vi "GUI.vi"() -> ()   [LabVIEW 2021]
doc: "The UDP protocol differs from TCP in that there is no error-checking with the packets of information that are sent, and thus no guarantee whatsoever that an intended recipient will actually receive a given piece of data.\n\nUDP does offer the ability to \"broadcast\" data across a network--simply specify an IP Address of all ones (255.255.255.255) to attempt to broadcast information network-wide. Keep in mind that routers and other network hardware will generally refuse to forward the broadcast beyond certain points, so the extent of the broadcast will in practice be limited."
panel:
  out "Waveform Chart":i32(graph)
  out "data out":string
  out "tx":i32
  in  "Stop":bool
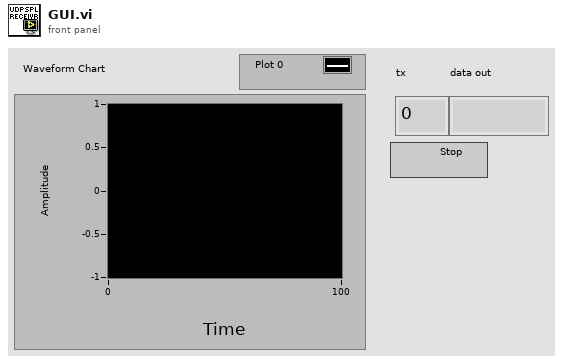
[diagram p1: front panel]
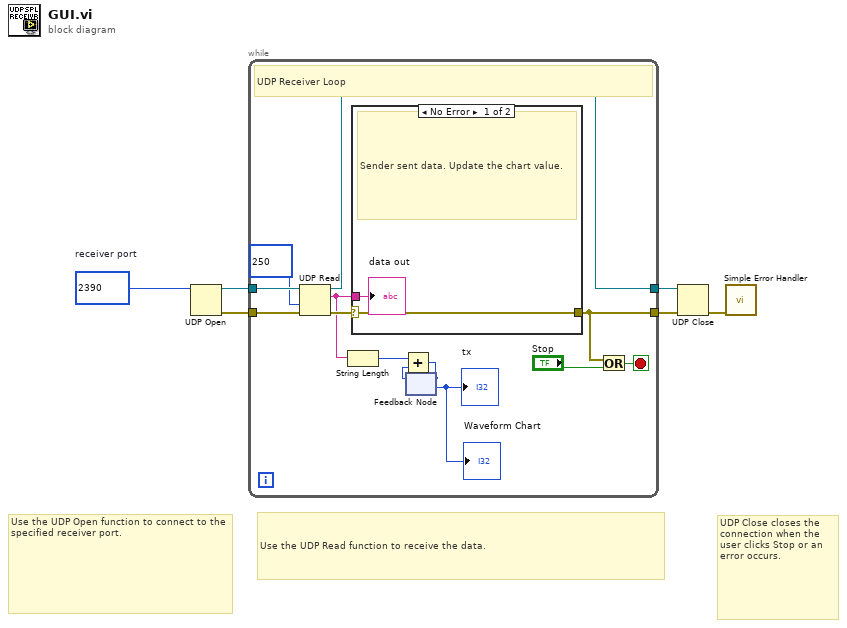
[diagram p0: block diagram]
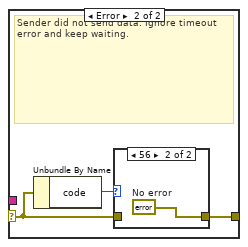
[diagram p2: hidden frame]
diagram:
  w1 = u16 2390  # receiver port
  # "UDP Close closes the connection when the user clicks Stop or an error occurs."
  # "Use the UDP Open function to connect to the specified receiver port."
  # "Use the UDP Read function to receive the data."
  n1 = UDP Open(11:w1) -> (port=w2:refnum<k16>, 0:w3:errorcluster)  [unwired: 4 in, 1 out]
  n2 = while {
    tunnel: w2 -> [w18]
    tunnel: [w11] -> w6
    tunnel: w3 -> [w15]
    tunnel: [w12] -> w4
    stop <- w16 stop-if-true
    # "UDP Receiver Loop"
    n3 = UDP Read(connection ID=w18, timeout ms (25000)=250, 8:w15) -> (data out=w10:string, error out=w13:errorcluster, 3:w11:refnum<k16>)  [unwired: 3 out]
    n4 = String Length(string=w10) -> (length=w9:i32)
    n5 = case shown="No Error" w13 {
      selector: w13 -> [w20 w22]
      tunnel: w10 -> [w19 _]
      tunnel: [w20 w21] -> w12
      frame No Error {
        # "Sender sent data. Update the chart value."
        "data out" <- w19
      }
      frame Error {
        # "Sender did not send data. Ignore timeout error and keep waiting."
        n6 = Unbundle By Name(w22) -> ("code"=w23:i32)
        n7 = case shown="56" w23 {
          tunnel: w22 -> [w24 _]
          tunnel: [w24 w25] -> w21
          frame Default {
          }
          frame 56 {
            w25 = errorcluster {"status"=FALSE, "code"=0, "source"=""}  # No error
          }
        }
      }
    }
    n8 = feedback #1() -> (w8:i32)  [unwired: 1 in]
    n9 = Add(x=w9, y=w8) -> (x+y=w7:i32)
    "tx" <- w7
    "Waveform Chart" <- w7
    n10 = feedback-in #1(w7) -> ()
    n11 = Or(x=w12, y="Stop") -> (x .or. y?=w16:bool)
  }
  n12 = UDP Close(connection ID=w6, 8:w4) -> (error out=w5:errorcluster)  [unwired: 1 out]
  n13 = call <vilib>:"Simple Error Handler.vi"("error in (no error)"=w5) -> ()  [unwired: 1 in, 8 out]
